vi "amp_dist.vi"() -> ()   [LabVIEW 2009]
panel:
  in  "増幅度":dbl
  in  "入力周波数(kHz)":dbl
  out "歪み率(%)":dbl
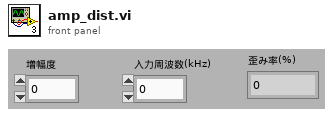
[diagram p1: front panel]
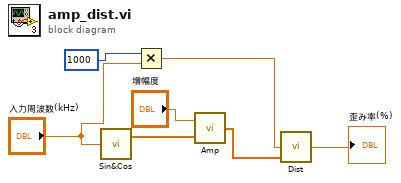
[diagram p0: block diagram]
diagram:
  n1 = call "Sin&Cos.vi"("周波数[kHz]"="入力周波数(kHz)") -> ("sin"=w7:dbl[])  [unwired: 1 out]
  n2 = Multiply(x=1000, y="入力周波数(kHz)") -> (x*y=w5:dbl)
  n3 = call "Amp.vi"("入力"=w7, "増幅率"="増幅度") -> ("出力"=w4:dbl[])
  n4 = call "Dist.vi"("入力"=w4, "基本周波数 [Hz]"=w5) -> ("ひずみ率"=→"歪み率(%)":dbl)  [unwired: 1 in]
